vi "Fixed Counter with FGV.vi"() -> ()   [LabVIEW 2012]
uses:
  Up Down Counter Command.ctl
panel:
  out "运行总数":i32
  in  "停止按钮":bool
  out "循环计数差":i32
  out "循环计数2":i32
  out "循环计数1":i32
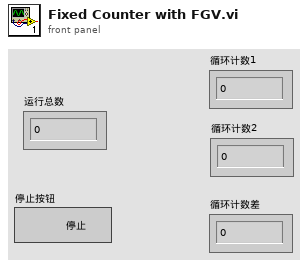
[diagram p1: front panel]
types:
  T1 = typedef "Up Down Counter Command.ctl" = enum16{"重置", "加1", "减1", "获取当前值"}
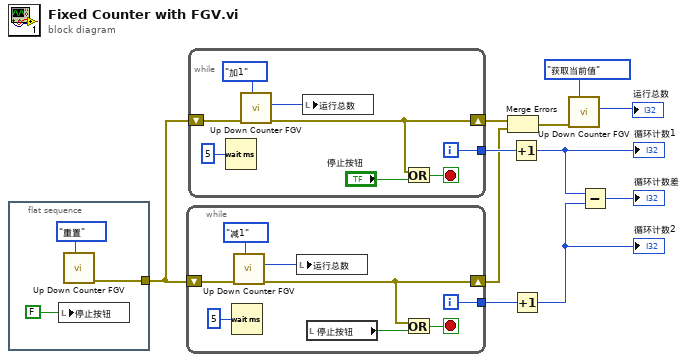
[diagram p0: block diagram]
diagram:
  n1 = flat-sequence {
    tunnel: [w12] -> w3
    frame #0 {
      n2 = local write "停止按钮"(FALSE ("停止按钮")) -> ()
      n3 = call "Up Down Counter FGV.vi"("操作选择"=Up_Down_Counter_Command."重置") -> ("错误输出"=w12:cluster{"状态":bool, "代码":i32, "源":string})  [unwired: 9 in, 1 out]
    }
  }
  n4 = while {
    tunnel: [w20] -> w10
    shift-right: [w15] -> w1
    shift-left: w3 -> [w17]
    i -> [w20]
    stop <- w16 stop-if-true
    n5 = Wait (ms) ("等待(ms)")(milliseconds to wait=u32 5 ("等待时间（毫秒）")) -> ()  [unwired: 1 out]
    n6 = call "Up Down Counter FGV.vi"("操作选择"=Up_Down_Counter_Command."减1", "错误输入"=w17) -> ("错误输出"=w15:cluster{"状态":bool, "代码":i32, "源":string}, "运行总数"=w19:i32)  [unwired: 8 in]
    n7 = local write "运行总数"(w19) -> ()
    n8 = local read "停止按钮"() -> (w22:bool)
    n9 = Or ("或")(x=w15, y=w22) -> (x .or. y?=w16:bool)
  }
  n10 = while {
    tunnel: [w28] -> w11
    shift-right: [w23] -> w6
    shift-left: w3 -> [w26]
    i -> [w28]
    stop <- w24 stop-if-true
    n11 = Wait (ms) ("等待(ms)")(milliseconds to wait=u32 5 ("等待时间（毫秒）")) -> ()  [unwired: 1 out]
    n12 = call "Up Down Counter FGV.vi"("操作选择"=Up_Down_Counter_Command."加1", "错误输入"=w26) -> ("错误输出"=w23:cluster{"状态":bool, "代码":i32, "源":string}, "运行总数"=w25:i32)  [unwired: 8 in]
    n13 = local write "运行总数"(w25) -> ()
    n14 = Or ("或")(x=w23, y="停止按钮") -> (x .or. y?=w24:bool)
  }
  n15 = Merge Errors ("合并错误")(w6, w1) -> (w2:errorcluster)
  n16 = Increment ("加1")(x=w11) -> (x+1=w9:i32)
  "循环计数1" <- w9
  n17 = Increment ("加1")(x=w10) -> (x+1=w8:i32)
  "循环计数2" <- w8
  n18 = call "Up Down Counter FGV.vi"("操作选择"=Up_Down_Counter_Command."获取当前值", "错误输入"=w2) -> ("运行总数"=→"运行总数":i32)  [unwired: 8 in, 1 out]
  n19 = Subtract ("减")(x=w9, y=w8) -> (x-y=→"循环计数差":i32)
